vi "SSL_get0_peername.vi"(8 "error in (no error)":errorcluster, 11 "SSL in":refnum<class "SSL.lvclass">) -> (0 "error out":errorcluster, 2 "Read bytes":string, 3 "SSL out":refnum<class "SSL.lvclass">)   [LabVIEW 2013, in "OpenSSL Socket.lvlib" / "SSL.lvclass"]
uses:
  SSL.lvclass
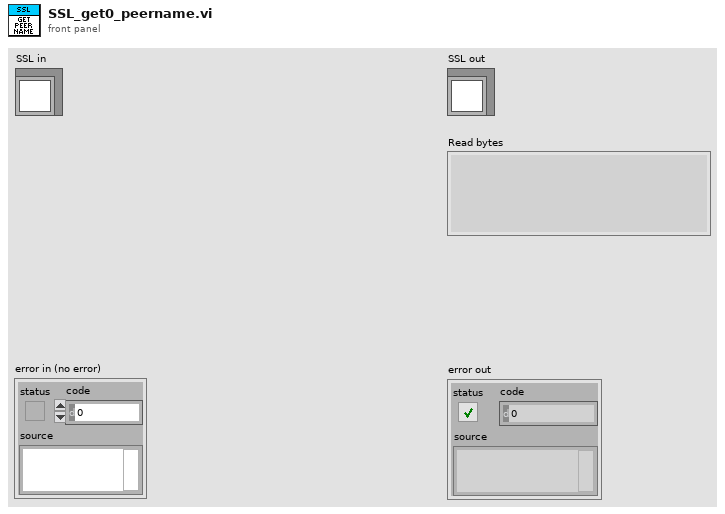
[diagram p1: front panel]
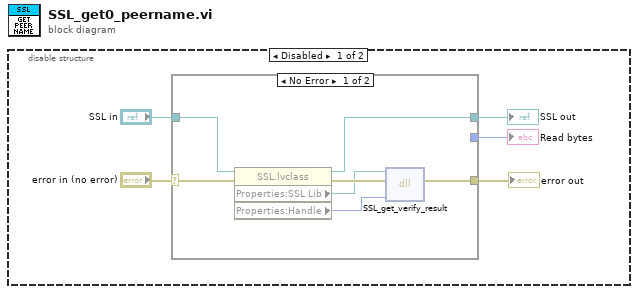
[diagram p0: block diagram]
diagram:
  n1 = disable-structure shown="Disabled" {
    frame Disabled {
      n2 = case shown="No Error" "error in (no error)" {
        selector: "error in (no error)" -> [w12 w13]
        tunnel: [w7 w14] -> w3
        tunnel: "SSL in" -> [w8 w14]
        tunnel: [w6 w13] -> w2
        tunnel: [_ _] -> w1
        frame No Error {
          n3 = property class="SSL.lvclass"(reference=w8, error in=w12) -> (reference out=w7:refnum<class "SSL.lvclass">, error out=w11:errorcluster, "Properties:SSL Lib"=w10:path, "Properties:Handle"=w9:u64)
          n4 = dll-call lib="C:/Program Files (x86)/National Instruments/Shared/nissl/NIssleay32.dll" fn="SSL_get_verify_result"(path in=w10, error in=w11, "SSL"=w9) -> (error out=w6:errorcluster)  [unwired: 3 in, 1 out]
        }
        frame Error {
        }
      }
      "SSL out" <- w3
      "error out" <- w2
      "Read bytes" <- w1
    }
    frame Enabled {
    }
  }
